vi "ASIC_ADC Read th.vi"(7 "Espera acceso FT":u32, 8 "error out 2":errorcluster, 10 "Sumador":u8, 11 "ftHandle_out 2":u32) -> (0 "error out":errorcluster, 1 "LLTH":dbl, 2 "HLTH":dbl, 3 "ftHandle_out":u32)   [LabVIEW 2009]
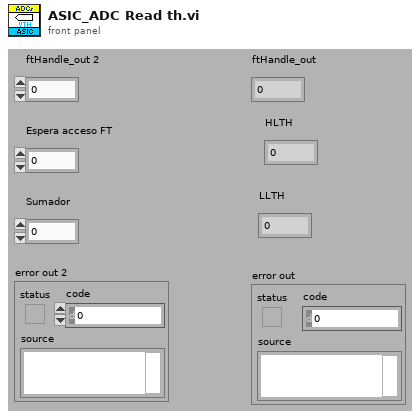
[diagram p1: front panel]
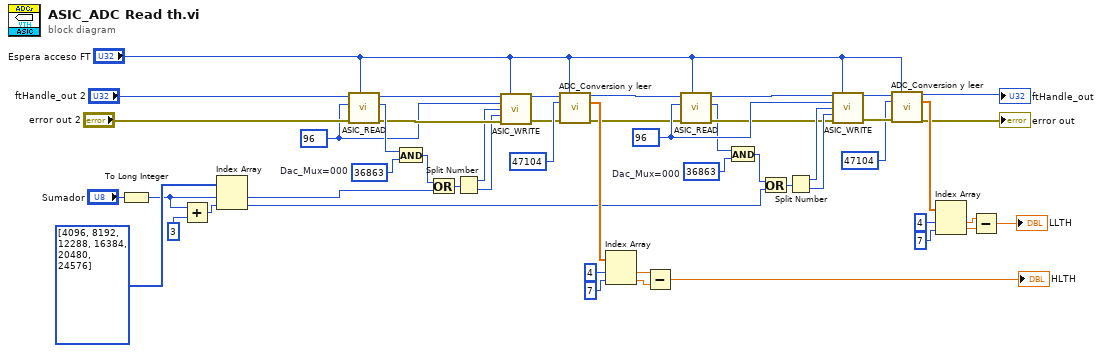
[diagram p0: block diagram]
diagram:
  w15 = u16 36863  # Dac_Mux=000
  w19 = u8 96 ("Direccion Registro Asic")
  w43 = u16 36863  # Dac_Mux=000
  w36 = u8 96 ("Direccion Registro Asic")
  n1 = To Long Integer(number="Sumador") -> (32bit integer=w40:i32)
  n2 = Add(x=w40, y=3) -> (x+y=w41:i32)
  n3 = Index Array(array=u16[] [4096, 8192, 12288, 16384, 20480, 24576], index #1=w40, index #2=w41) -> (element #1=w44:u16, element #2=w9:u16)
  n4 = call "ASIC_READ.vi"("Espera acceso USB"="Espera acceso FT", "error in"="error out 2", "Direccion Registro Asic"=w36, "ftHandle_in"="ftHandle_out 2") -> ("error out"=w37:errorcluster, "Valor Asic"=w47:u16, "ftHandle_out"=w38:u32)  [unwired: 5 in]
  n5 = And(x=w47, y=w43) -> (x .and. y?=w42:u16)
  n6 = Or(x=w42, y=w44) -> (x .or. y?=w35:u16)
  n7 = Split Number(x=w35) -> (hi(x)=w34:u8, lo(x)=w33:u8)
  n8 = call "ASIC_WRITE.vi"("ftHandle_in"=w38, "Espera acceso USB"="Espera acceso FT", "Direccion Registro Asic"=w36, "Byte Alto"=w34, "Byte Bajo"=w33, "error in"=w37) -> ("ftHandle_out"=w32:u32, "error out"=w31:errorcluster)  [unwired: 8 in]
  n9 = call "ADC_Conversion y leer.vi"("ftHandle_in 2"=w32, "Espera acceso USB"="Espera acceso FT", "Registro Conversion (0xD000)"=u16 47104, "error in 2"=w31) -> ("ftHandle_out"=w12:u32, "Datos Canal (V)"=w30:dbl[], "error out"=w11:errorcluster)  [unwired: 6 in, 3 out]
  n10 = Index Array(array=w30, index #1=4 ("index"), index #2=7 ("index")) -> (element #1=w3:dbl, element #2=w4:dbl)
  n11 = Subtract(x=w3, y=w4) -> (x-y=→"HLTH":dbl)
  n12 = call "ASIC_READ.vi"("Espera acceso USB"="Espera acceso FT", "error in"=w11, "Direccion Registro Asic"=w19, "ftHandle_in"=w12) -> ("error out"=w18:errorcluster, "Valor Asic"=w14:u16, "ftHandle_out"=w17:u32)  [unwired: 5 in]
  n13 = And(x=w14, y=w15) -> (x .and. y?=w16:u16)
  n14 = Or(x=w16, y=w9) -> (x .or. y?=w20:u16)
  n15 = Split Number(x=w20) -> (hi(x)=w21:u8, lo(x)=w22:u8)
  n16 = call "ASIC_WRITE.vi"("ftHandle_in"=w17, "Espera acceso USB"="Espera acceso FT", "Direccion Registro Asic"=w19, "Byte Alto"=w21, "Byte Bajo"=w22, "error in"=w18) -> ("ftHandle_out"=w23:u32, "error out"=w24:errorcluster)  [unwired: 8 in]
  n17 = call "ADC_Conversion y leer.vi"("ftHandle_in 2"=w23, "Espera acceso USB"="Espera acceso FT", "Registro Conversion (0xD000)"=u16 47104, "error in 2"=w24) -> ("ftHandle_out"=→"ftHandle_out":u32, "Datos Canal (V)"=w25:dbl[], "error out"=→"error out":errorcluster)  [unwired: 6 in, 3 out]
  n18 = Index Array(array=w25, index #1=4 ("index"), index #2=7 ("index")) -> (element #1=w6:dbl, element #2=w5:dbl)
  n19 = Subtract(x=w6, y=w5) -> (x-y=→"LLTH":dbl)
